vi "Initialization.vi"(8 "error in":errorcluster caption="error IO", 11 "VI Refnum":refnum<vi>) -> (0 "error out":errorcluster caption="error IO")   [LabVIEW 2019]
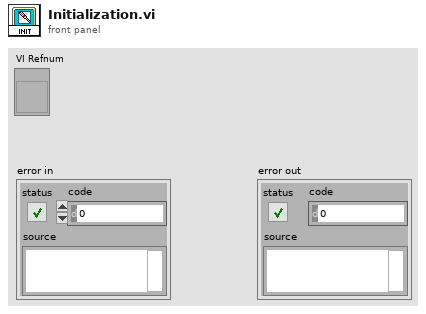
[diagram p1: front panel]
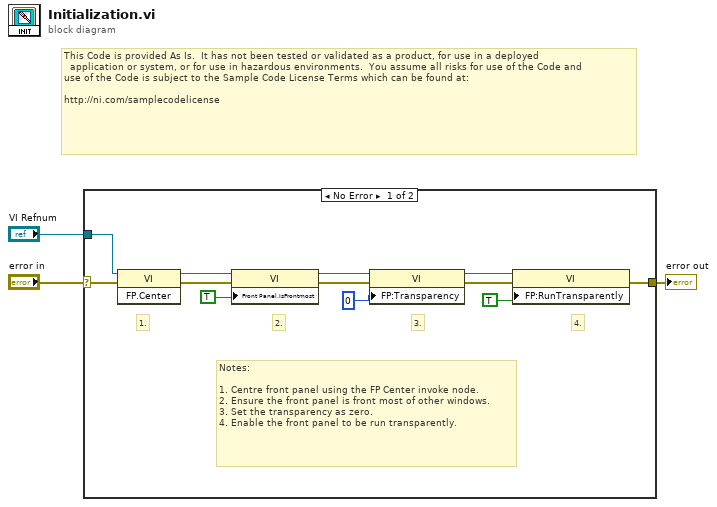
[diagram p0: block diagram]
diagram:
  # "This Code is provided As Is.  It has not been tested or validated as a product, for use in a deployed\n  application or system, or for use in hazardous environments.  You assume all risks for use of the Code and   \nuse of the Code is subject to the Sample Code License Terms which can be found at: \n\nhttp://ni.com/samplecodelicense"
  n1 = case shown="No Error" "error in" {
    selector: "error in" -> [w9 w16]
    tunnel: "VI Refnum" -> [w15 _]
    tunnel: [w10 w16] -> w1
    frame No Error {
      # "Notes:\n\n1. Centre front panel using the FP Center invoke node.\n2. Ensure the front panel is front most of other windows.\n3. Set the transparency as zero.\n4. Enable the front panel to be run transparently."
      # "4."
      # "3."
      # "2."
      # "1."
      n2 = invoke class="VI" method="FP.Center"(reference=w15, error in=w9) -> (reference out=w5:refnum<vi>, error out=w7:errorcluster)  [unwired: 1 in, 1 out]
      n3 = property class="VI"(reference=w5, error in=w7, "Front Panel.IsFrontmost"=TRUE ("Front Panel Window:Run VI Transparently")) -> (reference out=w4:refnum<vi>, error out=w6:errorcluster)
      n4 = property class="VI"(reference=w4, error in=w6, "FP:Transparency"=u8 0 ("Front Panel Window:Transparency")) -> (reference out=w11:refnum<vi>, error out=w12:errorcluster)
      n5 = property class="VI"(reference=w11, error in=w12, "FP:RunTransparently"=TRUE ("Front Panel Window:Run VI Transparently")) -> (error out=w10:errorcluster)  [unwired: 1 out]
    }
    frame Error {
    }
  }
  "error out" <- w1
